vi "RollerSpeed_Contactor.vi"() -> ()   [LabVIEW 2019]
uses:
  <vilib>/Instr/_visa.llb/VISA Configure Serial Port (Instr).vi
panel:
  out "BrakeTorque":sgl
  out "Current":sgl
  out "Voltage":sgl
  out "Speed Chart 2":dynamicdata(graph)
  out "Voltage/Current/Brake Chart":dynamicdata(graph)
  in  "t":sgl
  in  "test":bool
  out "WheelSpeed":sgl
  out "read buffer":string
  in  "?":bool
  out "RollerSpeed":sgl
  in  "VISA resource name":refnum<visa-resource-name>="COM5"
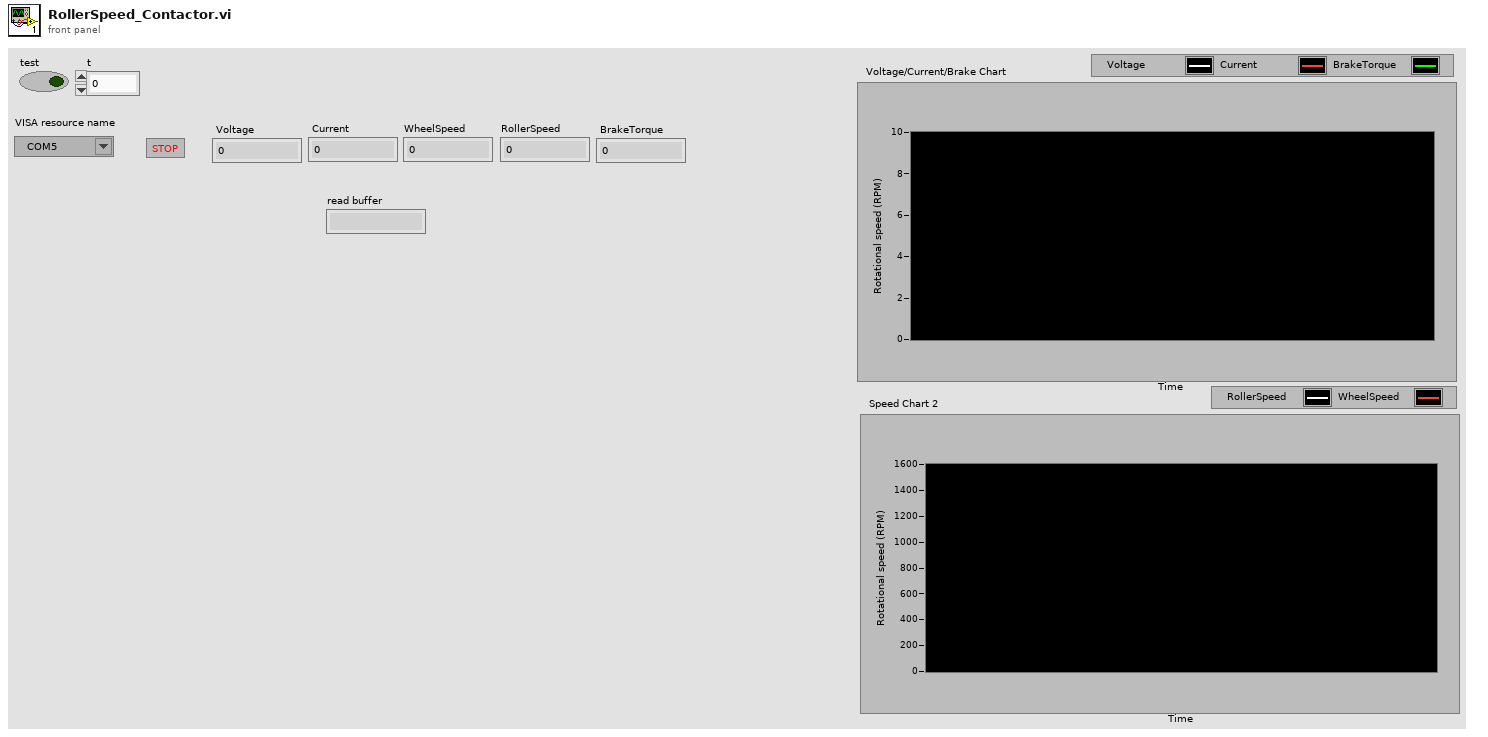
[diagram p1: front panel]
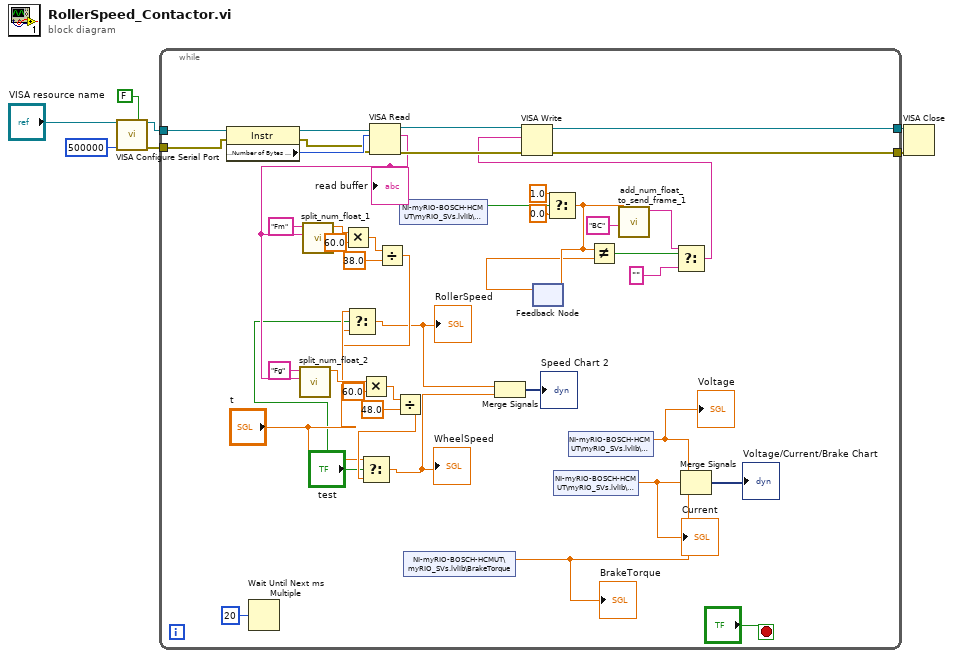
[diagram p0: block diagram]
diagram:
  n1 = call-poly "VISA Configure Serial Port"("VISA resource name"="VISA resource name", "Enable Termination\nChar (T)"=FALSE ("Enable Termination\nChar (T)"), "baud rate (9600)"=u32 500000) -> ("VISA resource name out"=w7:refnum<visa-resource-name>, "error out"=w6:errorcluster)  [unwired: 11 in]
  n2 = while {
    tunnel: w7 -> [w50]
    tunnel: w6 -> [w49]
    tunnel: [w43] -> w5
    tunnel: [w42] -> w4
    stop <- "?" stop-if-true
    n3 = property class="Instr"(reference=w50, error in=w49) -> (reference out=w48:refnum<visa-resource-name>, error out=w46:errorcluster, "Serial Settings:Number of Bytes at Serial Port"=w47:u32)
    n4 = Wait Until Next ms Multiple(millisecond multiple=u32 20) -> ()  [unwired: 1 out]
    n5 = VISA Read(VISA resource name=w48, byte count=w47, error in (no error)=w46) -> (VISA resource name out=w45:refnum<visa-resource-name>, read buffer=w19:string, error out=w44:errorcluster)  [unwired: 1 out]
    "read buffer" <- w19
    n6 = call "split_num_float_2.vi"("read_frame"=w19, "id (2 characters)"="Fg") -> ("num_float"=w21:sgl)  [unwired: 9 in]
    n7 = call "split_num_float_1.vi"("read_frame"=w19, "id (2 characters)"="Fm") -> ("num_float"=w36:sgl)  [unwired: 9 in]
    n8 = Multiply(x=w36, y=sgl 60.0) -> (x*y=w37:sgl)
    n9 = Multiply(x=w21, y=sgl 60.0) -> (x*y=w22:sgl)
    n10 = Divide(x=w37, y=sgl 38.0) -> (x/y=w16:sgl)
    n11 = Select(t="t", s="test", f=w16) -> (s? t:f=w12:sgl)
    "RollerSpeed" <- w12
    n12 = Divide(x=w22, y=sgl 48.0) -> (x/y=w18:sgl)
    n13 = Select(t="t", s="test", f=w18) -> (s? t:f=w11:sgl)
    "WheelSpeed" <- w11
    n14 = shared-variable "NI-myRIO-BOSCH-HCMUT\\myRIO_SVs.lvlib\\Boolean"() -> (w28:bool)  [unwired: 1 in, 1 out]
    n15 = shared-variable "NI-myRIO-BOSCH-HCMUT\\myRIO_SVs.lvlib\\BrakeTorque"() -> (w8:dbl)  [unwired: 1 in, 1 out]
    "BrakeTorque" <- w8
    n16 = Merge Signals(w12, w11) -> (→"Speed Chart 2":dynamicdata)
    n17 = feedback #1() -> (w25:sgl)  [unwired: 1 in]
    n18 = Select(t=sgl 1.0, s=w28, f=sgl 0.0) -> (s? t:f=w26:sgl)
    n19 = feedback-in #1(w26) -> ()
    n20 = shared-variable "NI-myRIO-BOSCH-HCMUT\\myRIO_SVs.lvlib\\Current"() -> (w9:dbl)  [unwired: 1 in, 1 out]
    "Current" <- w9
    n21 = shared-variable "NI-myRIO-BOSCH-HCMUT\\myRIO_SVs.lvlib\\Voltage"() -> (w10:dbl)  [unwired: 1 in, 1 out]
    "Voltage" <- w10
    n22 = Not Equal?(x=w26, y=w25) -> (x != y?=w27:bool)
    n23 = call "add_num_float_to_send_frame_1.vi"("num_float"=w26, "id (2 characters)"="BC") -> ("String"=w41:string)  [unwired: 9 in]
    n24 = Select(t=w41, s=w27, f="") -> (s? t:f=w40:string)
    n25 = VISA Write(VISA resource name=w45, write buffer=w40, error in (no error)=w44) -> (VISA resource name out=w42:refnum<visa-resource-name>, error out=w43:errorcluster)  [unwired: 1 out]
    n26 = Merge Signals(w10, w9, w8) -> (→"Voltage/Current/Brake Chart":dynamicdata)
  }
  n27 = VISA Close(VISA resource name=w4, error in (no error)=w5) -> ()  [unwired: 1 out]
